vi "Interface Read select.vi"(8 "error in (no error)":errorcluster, 9 "timeout":i32=10000, 10 "bytes to read":i32, 11 "interface in":refnum<class "Network Interface.lvclass">) -> (0 "error out":errorcluster, 1 "timed out?":bool, 2 "data":string, 3 "interface out":refnum<class "Network Interface.lvclass">)   [LabVIEW 2021, in "Network Interface.lvclass"]
doc: "This provides an interface for reading from a network bus."
uses:
  Network Interface.lvclass
  Network Interface.lvclass/Network Interface.ctl
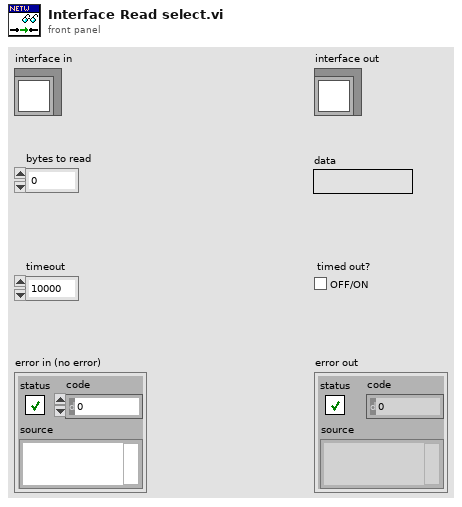
[diagram p1: front panel]
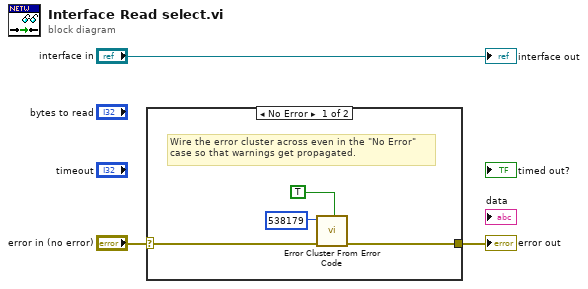
[diagram p0: block diagram]
diagram:
  n1 = case shown="No Error" "error in (no error)" {
    selector: "error in (no error)" -> [w6 w8]
    tunnel: [w5 w8] -> w2
    frame No Error {
      # "Wire the error cluster across even in the \"No Error\"\ncase so that warnings get propagated."
      n2 = call <vilib>:"Error Cluster From Error Code.vi"("is warning? (False)"=TRUE ("show call chain? (False)"), "error in (no error)"=w6, "error code (0)"=538179) -> ("error out"=w5:errorcluster)  [unwired: 6 in]
    }
    frame Error {
    }
  }
  "error out" <- w2
  "interface out" <- "interface in"
